vi "Test_Load Folder Map.vi"() -> ()   [LabVIEW 2019]
uses:
  Ctl/Ctl_Config_Folder Icon Map.ctl
  <vilib>/Utility/config.llb/NI_LVConfig.lvlib
  AutoMenuCreator.lvlib
panel:
  out "Folder Icon Map":T1
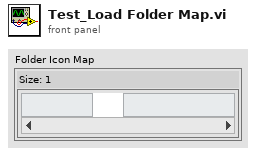
[diagram p1: front panel]
types:
  T1 = typedef "AutoMenuCreator.lvlib/Ctl_Config_Folder Icon Map.ctl" = map{string, path}
  T2 = typedef "NI_LVConfig.lvlib/Config Data RefNum.ctl" = refnum<k1>
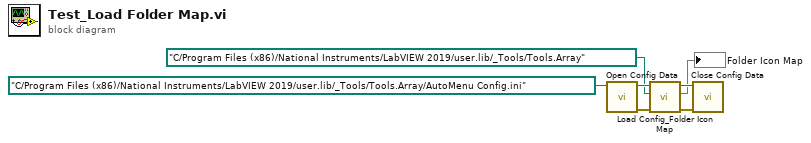
[diagram p0: block diagram]
diagram:
  n1 = call <vilib>:"Open Config Data.vi"("configuration file path"=path "C:/Program Files (x86)/National Instruments/LabVIEW 2019/user.lib/_Tools/Tools.Array/AutoMenu Config.ini") -> ("error out"=w6:errorcluster, "refnum"=w7:T2)  [unwired: 8 in, 1 out]
  n2 = call "Load Config_Folder Icon Map.vi"("error in (no error)"=w6, "Target Folder"=path "C:/Program Files (x86)/National Instruments/LabVIEW 2019/user.lib/_Tools/Tools.Array", "Refnum in"=w7) -> ("error out"=w4:errorcluster, "Folder Icon Map"=→"Folder Icon Map":T1, "Refnum out"=w5:T2)  [unwired: 6 in]
  n3 = call <vilib>:"Close Config Data.vi"("error in (no error)"=w4, "refnum"=w5) -> ()  [unwired: 8 in, 2 out]
